vi "Graphics Folder.vi"() -> (1 "Graphics Folder":path)   [LabVIEW 2020, in "VolatusGUIControls.lvlib"]
uses:
  VolatusGUIControls.lvlib
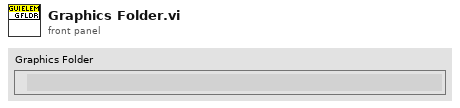
[diagram p1: front panel]
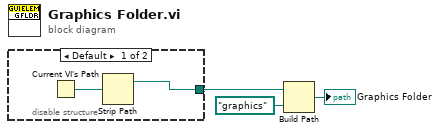
[diagram p0: block diagram]
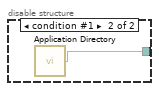
[diagram p2: hidden frame]
diagram:
  n1 = disable-structure shown="Default" {
    disable-tunnel: [w4 w6] -> w2
    frame condition #0 (active) {
      n2 = Current VI's Path() -> (path=w5:path)
      n3 = Strip Path(path=w5) -> (stripped path=w4:path)  [unwired: 1 out]
    }
    frame condition #1 {
      n4 = call <vilib>:"Application Directory.vi"() -> ("Application Directory"=w6:path)
    }
  }
  n5 = Build Path(base path=w2, name or relative path=path "graphics") -> (appended path=→"Graphics Folder":path)
